vi "average sensor reading.vi"() -> ()   [LabVIEW 2018]
panel:
  out "Avg values":dbl[](array[numeric])
  in  "Sensor values":dbl
  in  "?":bool
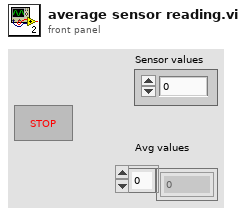
[diagram p1: front panel]
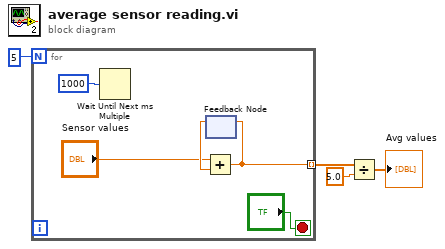
[diagram p0: block diagram]
diagram:
  n1 = for {
    N: 5 -> [_]
    tunnel: [w6] -> w1 mode=indexing
    stop <- "?" stop-if-true
    n2 = Wait Until Next ms Multiple(millisecond multiple=u32 1000) -> ()  [unwired: 1 out]
    n3 = feedback #1() -> (w9:dbl)  [unwired: 1 in]
    n4 = Add(x="Sensor values", y=w9) -> (x+y=w6:dbl)
    n5 = feedback-in #1(w6) -> ()
  }
  n6 = Divide(x=w1, y=5.0) -> (x/y=→"Avg values":dbl[])
